vi "LIDAR Line mux test bench.vi"() -> ()   [LabVIEW 2011]
panel:
  out "Data Aquired 2":picture
  out "Data Aquired":picture
  in  "Max Distance":dbl=3000.0 format="%0.2f"
  in  "Direction":dbl[](array[numeric])
  in  "Magnitude":dbl[](array[numeric])
  in  "Line Data":T1(array[cluster])
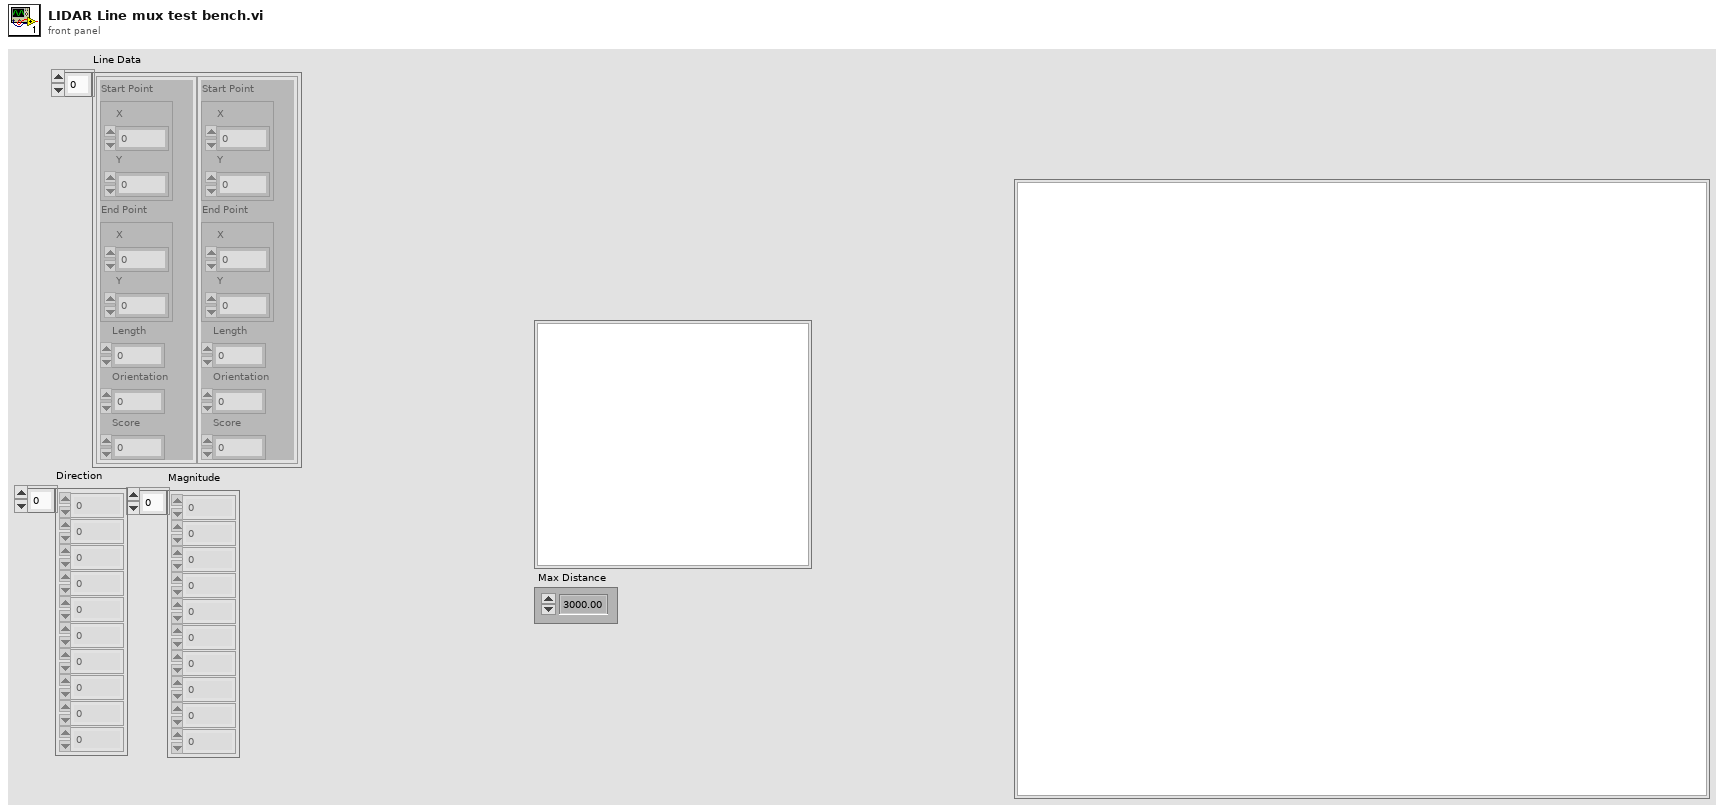
[diagram p1: front panel]
types:
  T1 = cluster{"Start Point":cluster{"X":sgl, "Y":sgl}, "End Point":cluster{"X":sgl, "Y":sgl}, "Length":dbl, "Orientation":dbl, "Score":dbl}[]
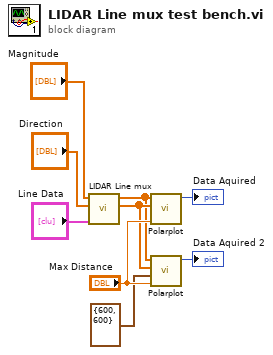
[diagram p0: block diagram]
diagram:
  n1 = call "LIDAR Line mux.vi"("Lines In"="Line Data", "Angle In"="Direction", "Range In"="Magnitude") -> ("Angle Out"=w2:dbl[], "Range Out"=w1:dbl[])  [unwired: 7 in]
  n2 = call "Polarplot.vi"("maximum"="Max Distance", "Direction"=w2, "Magnitude"=w1) -> ("Data Aquired"=→"Data Aquired":picture)  [unwired: 8 in]
  n3 = call "Polarplot.vi"("maximum"="Max Distance", "dimensions (w,h)"=cluster{"width":i16, "height":i16} {"width"=600, "height"=600}, "Direction"=w2, "Magnitude"=w1) -> ("Data Aquired"=→"Data Aquired 2":picture)  [unwired: 7 in]
